vi "Post-Install Custom Action.vi"(10 "Variant":variant) -> (0 "error out":errorcluster)   [LabVIEW 2020]
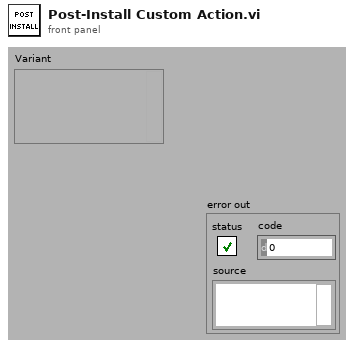
[diagram p1: front panel]
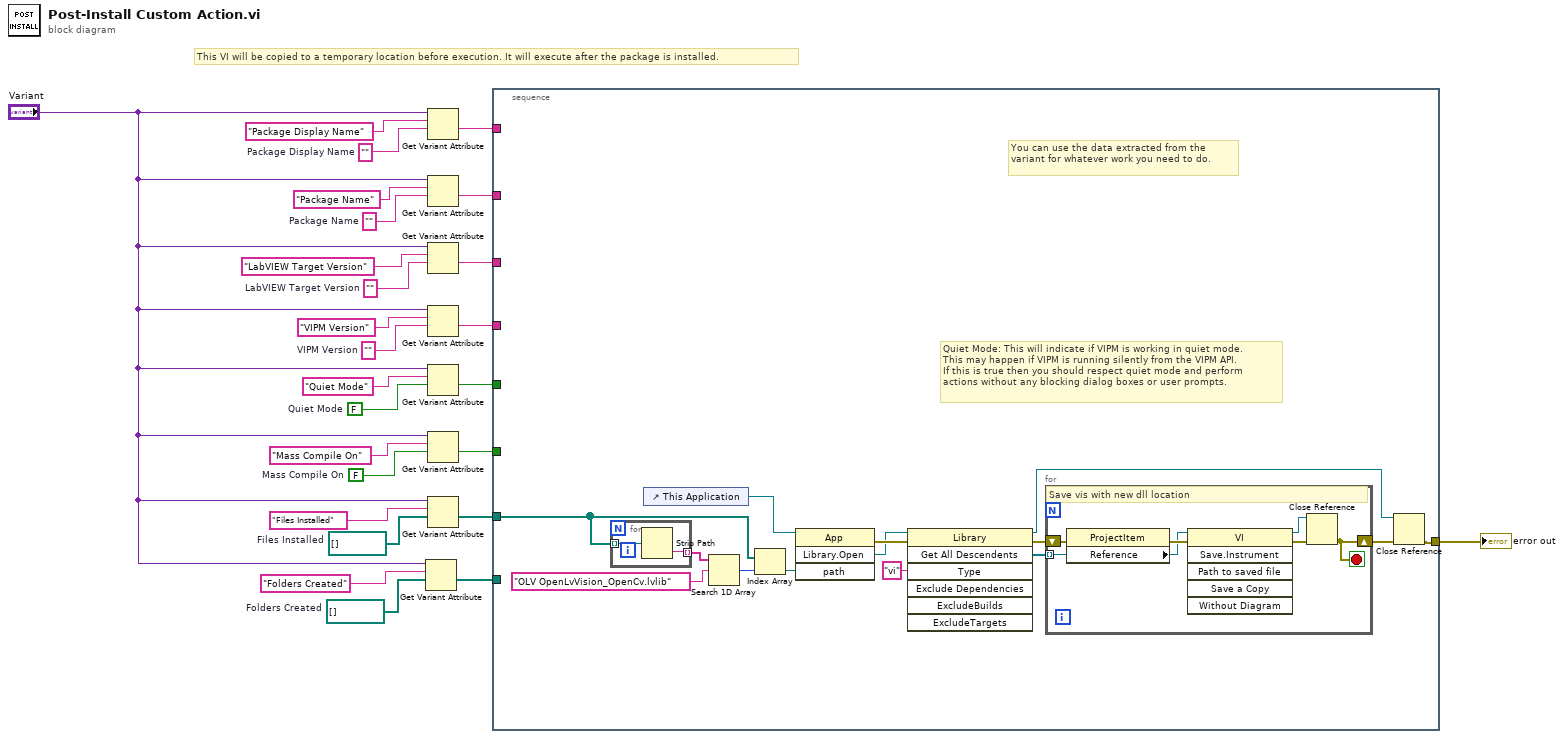
[diagram p0: block diagram]
diagram:
  w2 = path[] []  # Folders Created
  w3 = path[] []  # Files Installed
  w9 = FALSE  # Mass Compile On
  w10 = ""  # Package Display Name
  w17 = FALSE  # Quiet Mode
  w20 = ""  # VIPM Version
  w22 = ""  # LabVIEW Target Version
  w24 = ""  # Package Name
  # "This VI will be copied to a temporary location before execution. It will execute after the package is installed."
  n1 = Get Variant Attribute(Variant="Variant", name="Folders Created", default value (empty Variant)=w2) -> (value=w7:path[])  [unwired: 1 in, 3 out]
  n2 = Get Variant Attribute(Variant="Variant", name="Package Display Name", default value (empty Variant)=w10) -> (value=w16:string)  [unwired: 1 in, 3 out]
  n3 = Get Variant Attribute(Variant="Variant", name="Package Name", default value (empty Variant)=w24) -> (value=w15:string)  [unwired: 1 in, 3 out]
  n4 = Get Variant Attribute(Variant="Variant", name="LabVIEW Target Version", default value (empty Variant)=w22) -> (value=w14:string)  [unwired: 1 in, 3 out]
  n5 = Get Variant Attribute(Variant="Variant", name="VIPM Version", default value (empty Variant)=w20) -> (value=w13:string)  [unwired: 1 in, 3 out]
  n6 = Get Variant Attribute(Variant="Variant", name="Quiet Mode", default value (empty Variant)=w17) -> (value=w12:bool)  [unwired: 1 in, 3 out]
  n7 = Get Variant Attribute(Variant="Variant", name="Mass Compile On", default value (empty Variant)=w9) -> (value=w11:bool)  [unwired: 1 in, 3 out]
  n8 = Get Variant Attribute(Variant="Variant", name="Files Installed", default value (empty Variant)=w3) -> (value=w6:path[])  [unwired: 1 in, 3 out]
  n9 = stacked-sequence {
    tunnel: w16 -> [_]
    tunnel: w15 -> [_]
    tunnel: w14 -> [_]
    tunnel: w13 -> [_]
    tunnel: w12 -> [_]
    tunnel: w11 -> [_]
    tunnel: w6 -> [w30]
    tunnel: w7 -> [_]
    tunnel: [w27] -> w1
    frame #0 {
      # "Quiet Mode: This will indicate if VIPM is working in quiet mode.\nThis may happen if VIPM is running silently from the VIPM API.\nIf this is true then you should respect quiet mode and perform\nactions without any blocking dialog boxes or user prompts."
      # "You can use the data extracted from the variant for whatever work you need to do."
      n10 = for {
        tunnel: w30 -> [w41] mode=indexing
        tunnel: [w42] -> w32 mode=indexing
        n11 = Strip Path(path=w41) -> (name=w42:string)  [unwired: 1 out]
      }
      n12 = control-ref of="This Application"() -> (w33:refnum<vi>)
      n13 = Search 1D Array(1D array=w32, element="OLV OpenLvVision_OpenCv.lvlib") -> (index of element=w31:i32)  [unwired: 1 in]
      n14 = Index Array(array=w30, index=w31) -> (element=w29:path)
      n15 = invoke class="App" method="Library.Open"(reference=w33, "path"=w29) -> (error out=w37:errorcluster, "Open Library"=w36:refnum<vi>)  [unwired: 2 in, 2 out]
      n16 = invoke class="Library" method="Get All Descendents"(reference=w36, error in=w37, "Type"="vi") -> (reference out=w34:refnum<vi>, error out=w38:errorcluster, "All Descendents"=w40:refnum<vi>[])  [unwired: 4 in, 4 out]
      n17 = for {
        tunnel: w40 -> [w49] mode=indexing
        shift-right: [w43] -> w35
        shift-left: w38 -> [w46]
        stop <- w43 stop-if-true
        # "Save vis with new dll location"
        n18 = property class="ProjectItem"(reference=w49, error in=w46) -> (error out=w48:errorcluster, "Reference"=w47:refnum<vi>)  [unwired: 1 out]
        n19 = invoke class="VI" method="Save.Instrument"(reference=w47, error in=w48) -> (reference out=w44:refnum<vi>, error out=w45:errorcluster)  [unwired: 4 in, 4 out]
        n20 = Close Reference(reference=w44, error in (no error)=w45) -> (error out=w43:errorcluster)
      }
      n21 = Close Reference(reference=w34, error in (no error)=w35) -> (error out=w27:errorcluster)
    }
  }
  "error out" <- w1
